vi "Get all descriptions in project.vi"(7 "Folder Path":path=path "V:/Oslo/xg237/170606_xg237_wind_chromatin_1" caption="Root path") -> (1 "All descriptions":string="Trace_0000_Oscilloscope\\description: Initialization and oscilloscope data go here\r\nTrace_0014\\description: good 1\r\nTrace_0019\\description: good 2\r\nTrace_0037\\description: good 3\r\nTrace_0038\\description: good 4 braiding?\r\nTrace_0039\\description: good 4 braiding?\r\nTrace_0044\\description: good 5\r\nTrace_0049\\description: good 6-1\r\nTrace_0050\\description: good 6-2\r\nTrace_0053\\description: good 6-3 cannot achieve last step!!!\r\nTrace_0054\\description: error\r\nTrace_0058\\description: good 6-4 whole\r\nTrace_0059\\description: good 6-5 nucleosome depleted\r\nTrace_0060\\description: good 6-6 nucleosome depleted\r\nTrace_0061\\description: good 6-7 nucleosome depleted\r\nTrace_0062\\description: good 7 non-tc but stretching is good\r\nTrace_0067\\description: good ? 8\r\nTrace_0068\\description: good but break in the middle!\r\nTrace_0069\\description: good but break in the middle!\r\nTrace_0070\\description: braiding?\r\nTrace_0075\\description: good 9 1st multiple winding\r\nTrace_0082\\description: good but break in the middle 10\r\nTrace_0083\\description: good but break in the middle 11\r\nTrace_0086\\description: good weird?\r\nTrace_0092\\description: good only first trace sqeeze the nucleosome out\r\nTrace_0095\\description: good 12 only whole curve got\r\n", 2 "Descriptions and trace index":cluster{i32[], string[]})   [LabVIEW 2020]
uses:
  BasicVIs/BasicVIs.lvlib
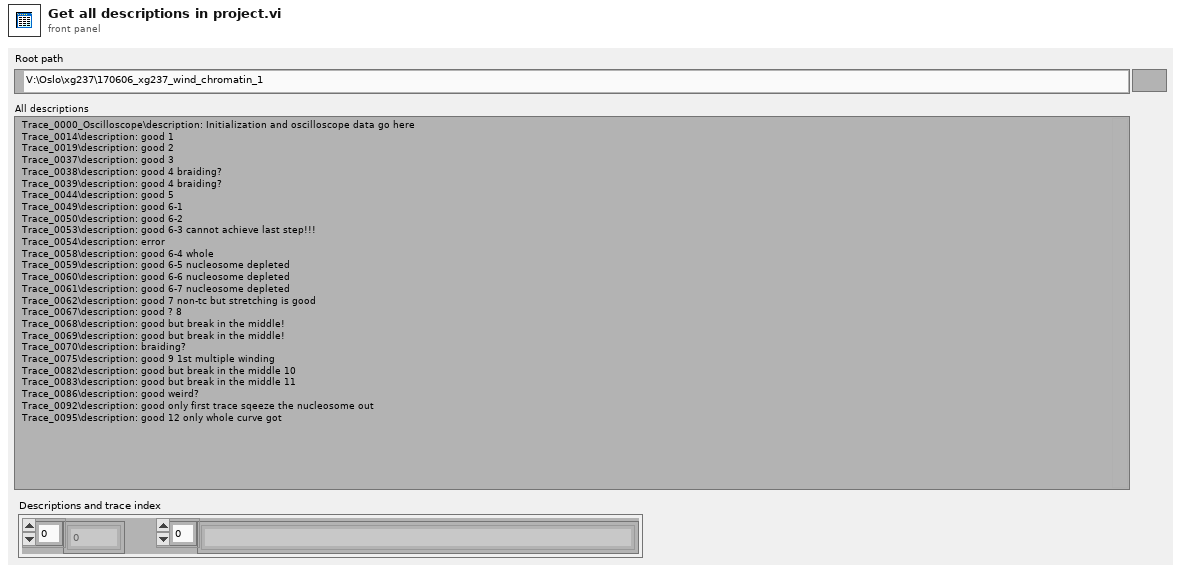
[diagram p1: front panel]
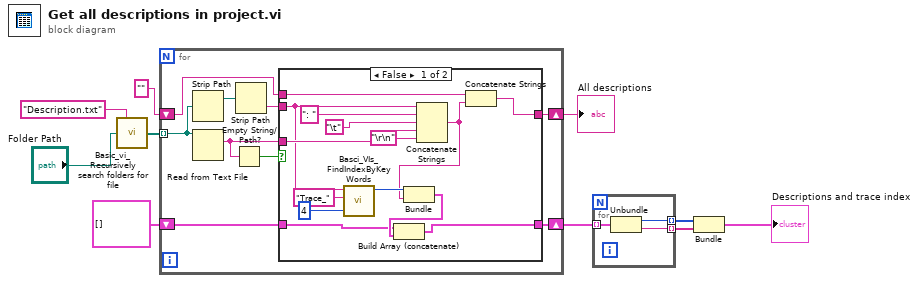
[diagram p0: block diagram]
diagram:
  n1 = call "Basic_vi_Recursively search folders for file.vi"("File name"="Description.txt", "Folder Path"="Folder Path") -> ("All folders containing .txt and .bin files"=w7:path[])  [unwired: 13 in]
  n2 = for {
    tunnel: w7 -> [w14] mode=indexing
    shift-right: [w18] -> w9
    shift-left: "" ("String") -> [w19]
    shift-right: [w11] -> w2
    shift-left: cluster{"Folder index":i32, string}[] [] -> [w12]
    n3 = Strip Path(path=w14) -> (stripped path=w15:path)  [unwired: 1 out]
    n4 = Read from Text File(file (use dialog)=w14) -> (text=w17:string)  [unwired: 3 in, 3 out]
    n5 = Empty String/Path?(string/path=w17) -> (empty?=w16:bool)
    n6 = Strip Path(path=w15) -> (name=w13:string)  [unwired: 1 out]
    n7 = case shown="False" w16 {
      tunnel: w17 -> [w24 _]
      tunnel: w19 -> [w33 w35]
      tunnel: [w26 w35] -> w18
      tunnel: w13 -> [w21 _]
      tunnel: w12 -> [w28 w34]
      tunnel: [w27 w34] -> w11
      frame False {
        n8 = call "Basci_VIs_FindIndexByKeyWords.vi"("Max length\nof index"=4 ("Max length\nof index"), "Key words"="Trace_", "String input"=w21) -> ("Folder index"=w30:i32)  [unwired: 1 in, 3 out]
        n9 = Concatenate Strings(w21, ": " ("string"), "\t", w24, "\r\n") -> (w20:string)
        n10 = Bundle("Folder index"=w30, w20) -> (w29:cluster{"Folder index":i32, string})  [unwired: 1 in]
        n11 = Build Array (concatenate)(w28, w29) -> (w27:cluster{"Folder index":i32, string}[])
        n12 = Concatenate Strings(w33, w20) -> (w26:string)
      }
      frame True {
      }
    }
  }
  "All descriptions" <- w9
  n13 = for {
    tunnel: w2 -> [w38] mode=indexing
    tunnel: [w37] -> w4 mode=indexing
    tunnel: [w36] -> w3 mode=indexing
    n14 = Unbundle(w38) -> ("Folder index"=w37:i32, w36:string)
  }
  n15 = Bundle(w4, w3) -> (→"Descriptions and trace index":cluster{i32[], string[]})  [unwired: 1 in]
